vi "Example.vi"() -> ()   [LabVIEW 2017]
uses:
  Source/LAChatByText.vi
  Source/LAOnMessage.vi
  Source/LAOnChunk.vi
  Source/LAOnFunctionCall.vi
  Source/LAOnDone.vi
  Source/LAOnError.vi
  LiteAgentSDK.lvlib
panel:
  out "ToolReturn":cluster{"id":string, "result":variant}
  out "FunctionCall":T1
  out "AgentMessageChunkCompletions":T2
  out "AgentMessageChunkPart":T3
  out "AgentMessageChunkCommon":T4
  out "AgentMessageCompletions":T2
  out "AgentMessageContent":T5
  out "AgentMessageCommon":T4
  in  "Error In":errorcluster
  out "Error Output":errorcluster caption="Error Out"
  out "SessionId":string
  out "Version":string
  out "EventMessages":string
  out "Prompt":string
  out "AgentId":string
  out "ApiKey":string
  out "BaseUrl":string
  # "AgentMessage"
  # "AgentMessageChunk"
  # "FunctionCall & ToolReturn"
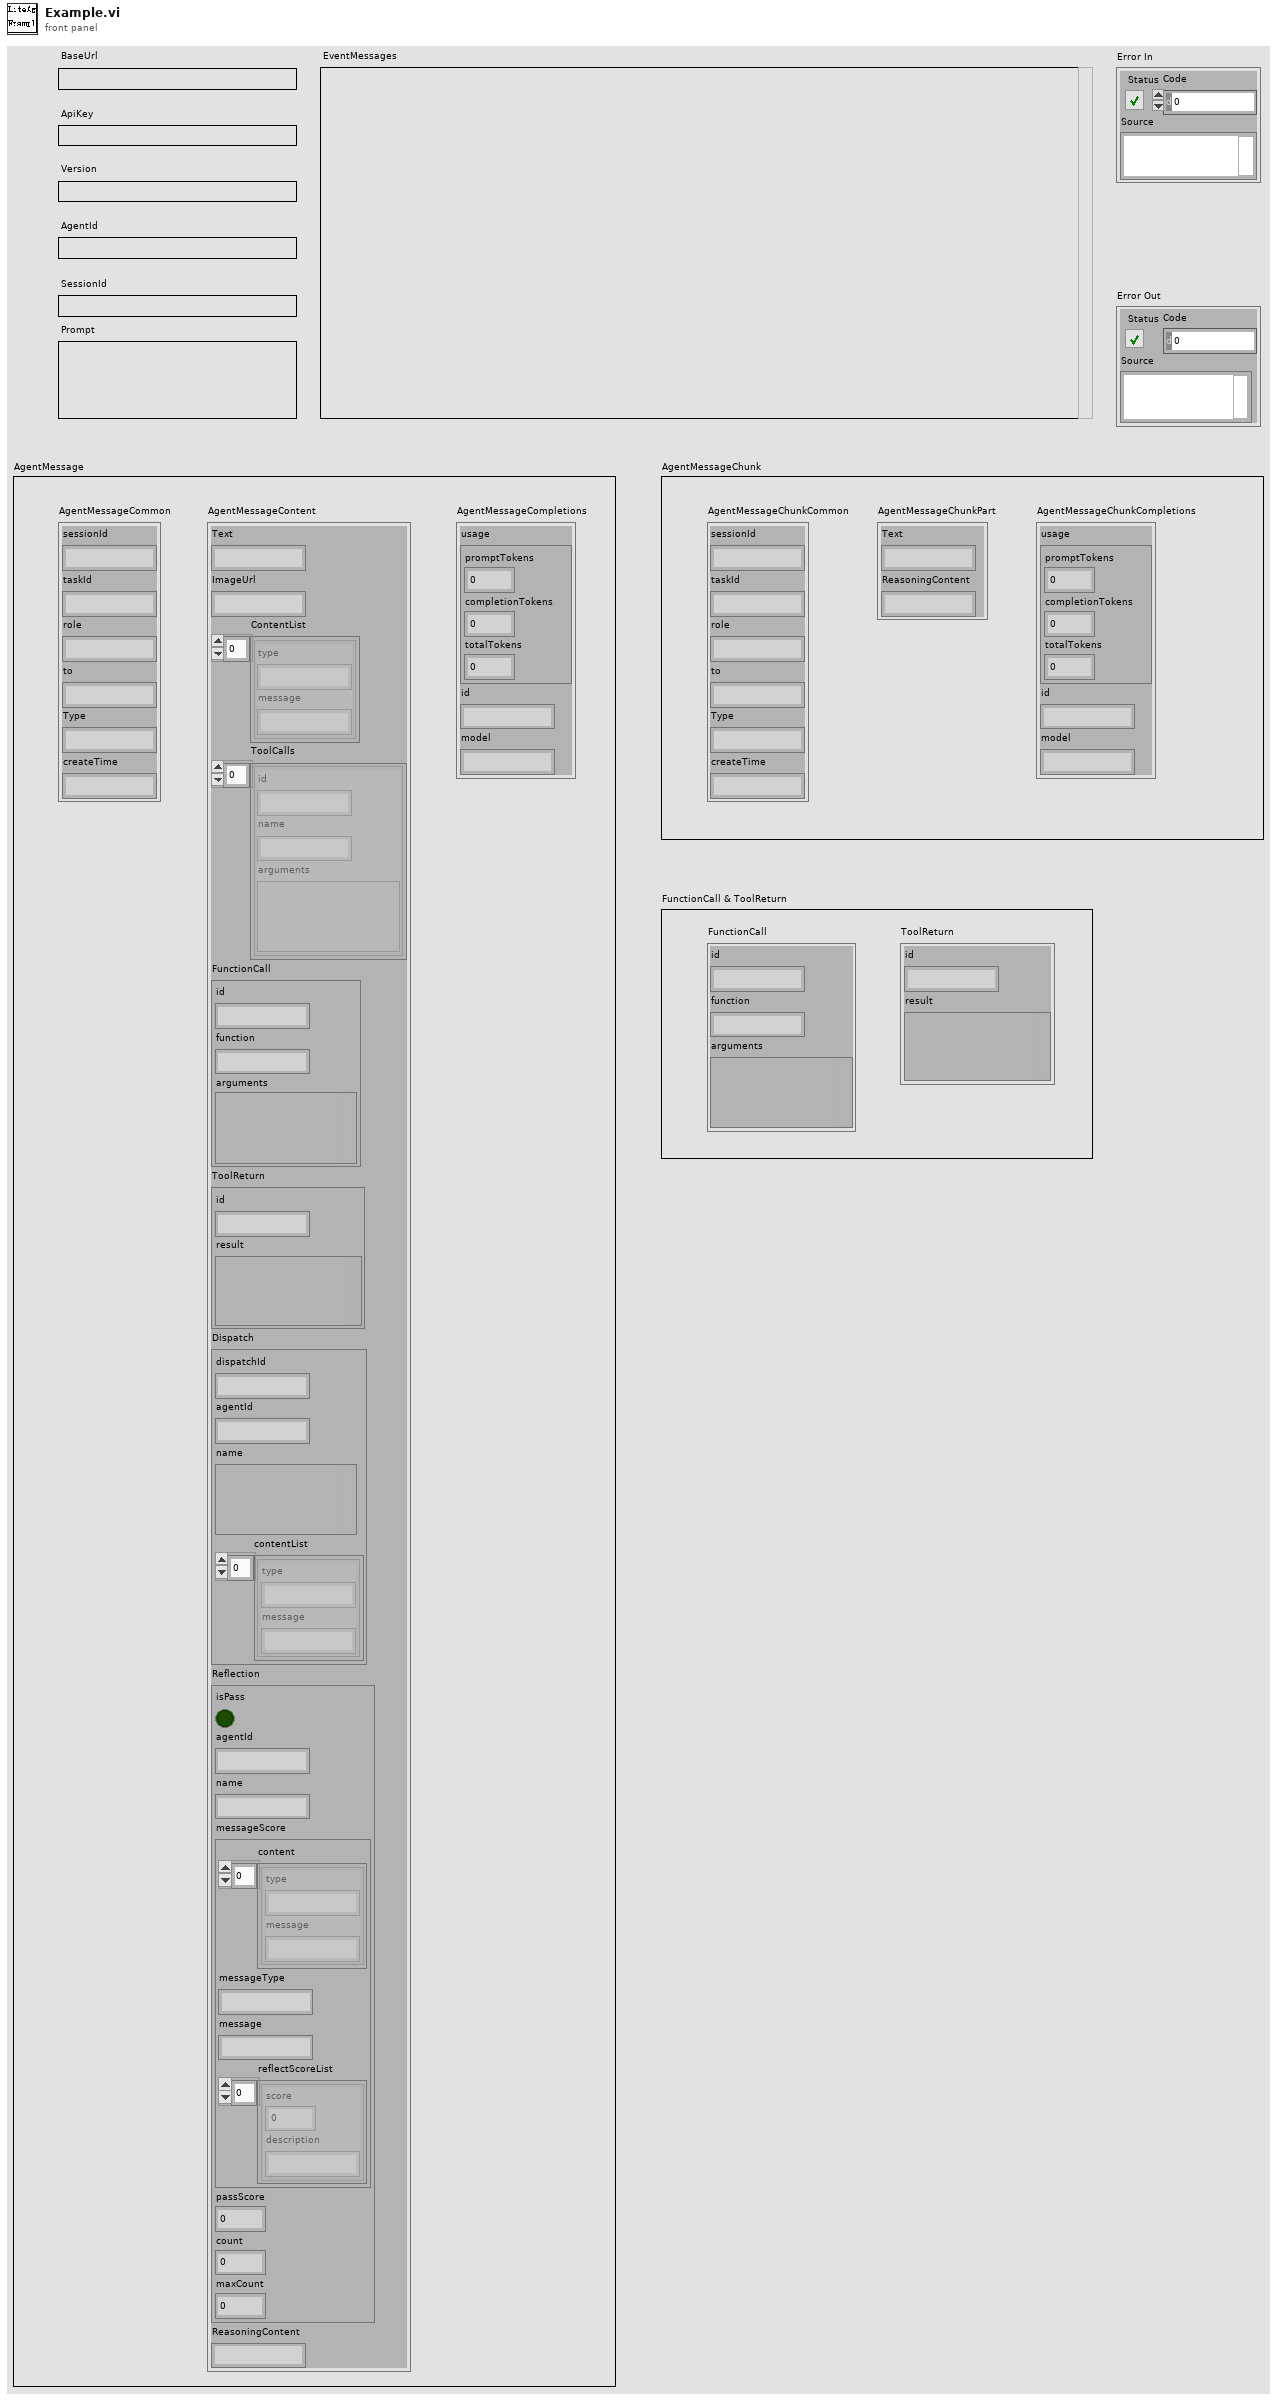
[diagram p1: front panel]
types:
  T1 = cluster{"id":string, "function":string, "arguments":variant}
  T2 = cluster{"usage":cluster{"promptTokens":i32, "completionTokens":i32, "totalTokens":i32}, "id":string, "model":string}
  T3 = cluster{"Text":string, "ReasoningContent":string}
  T4 = cluster{"sessionId":string, "taskId":string, "role":string, "to":string, "Type":string, "createTime":string}
  T5 = cluster{"Text":string, "ImageUrl":string, "ContentList":cluster{"type":string, "message":string}[], "ToolCalls":cluster{"id":string, "name":string, "arguments":variant}[], "FunctionCall":cluster{"id":string, "function":string, "arguments":variant}, "ToolReturn":cluster{"id":string, "result":variant}, "Dispatch":cluster{"dispatchId":string, "agentId":string, "name":variant, "contentList":cluster{"type":string, "message":string}[]}, "Reflection":cluster{"isPass":bool, "agentId":string, "name":string, "messageScore":cluster{"content":cluster{"type":string, "message":string}[], "messageType":string, "message":string, "reflectScoreList":cluster{"score":i32, "description":string}[]}, "passScore":i32, "count":i32, "maxCount":i32}, "ReasoningContent":string}
  T6 = cluster{"BaseUrl":string, "ApiKey":string, "LiteAgentSDK":refnum<k24>, "AgentId":string, "SessionId":string, "OnEventQueue":refnum<queue>, "CurrEventJson":variant}
  T7 = cluster{"sessionId":string, "taskId":string, "role":string, "to":string, "type":string, "content":variant, "completions":variant, "createTime":string}
  T8 = cluster{"sessionId":string, "taskId":string, "role":string, "to":string, "type":string, "part":variant, "completions":variant, "createTime":string}
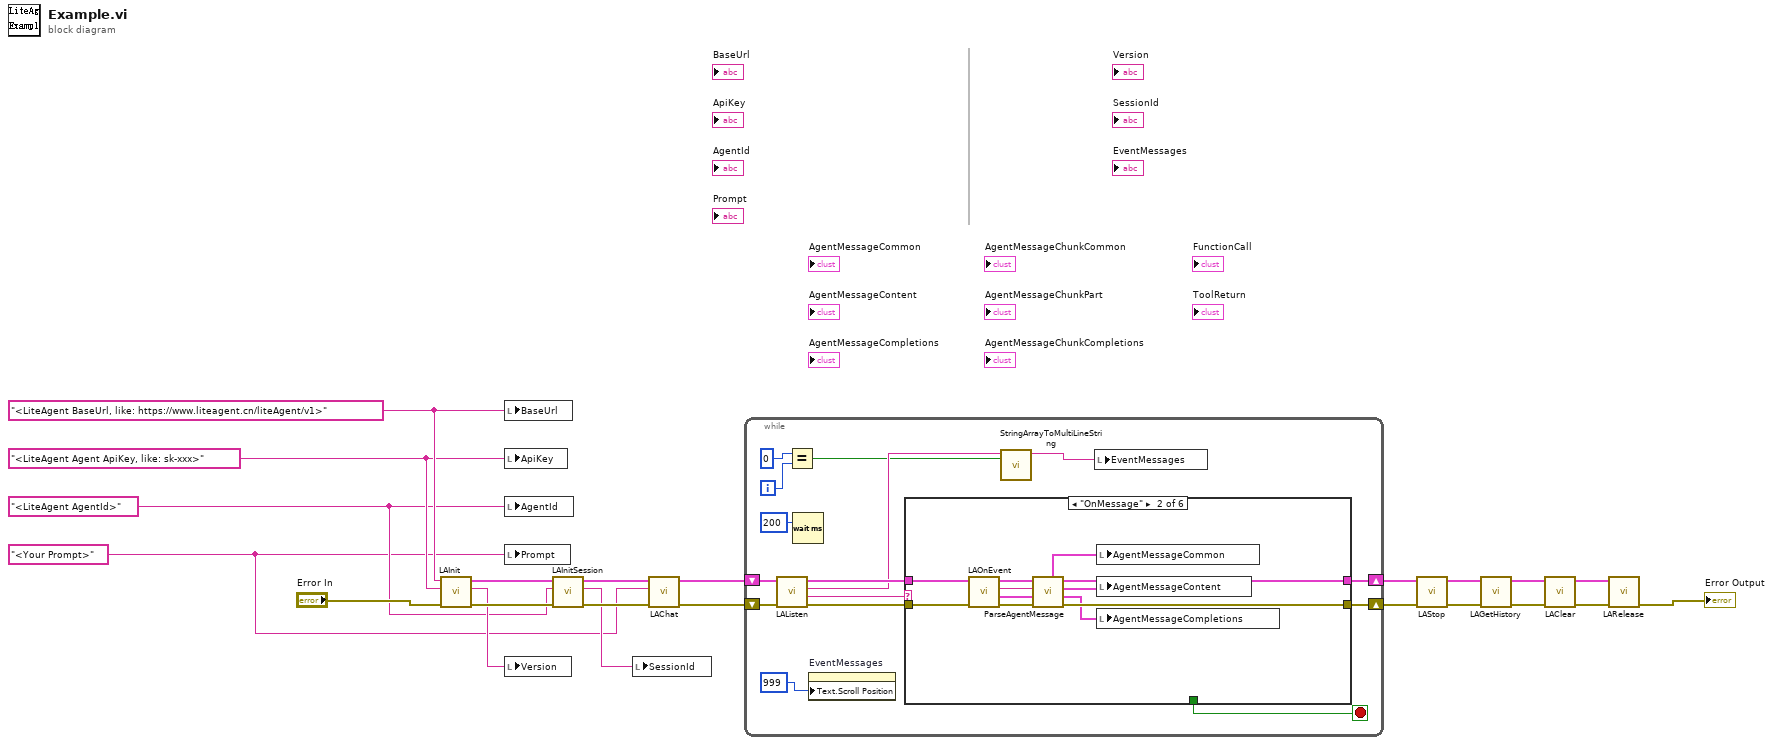
[diagram p0: block diagram]
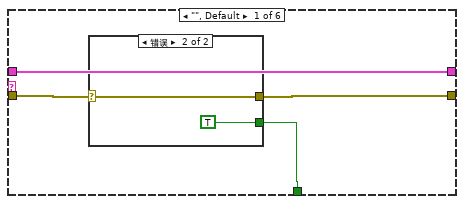
[diagram p2: hidden frame]
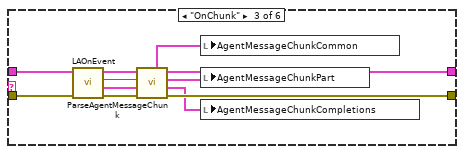
[diagram p4: hidden frame]
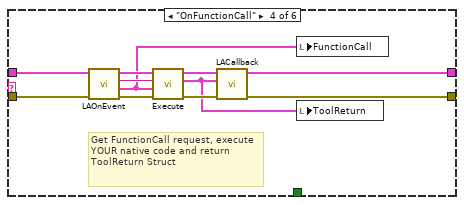
[diagram p5: hidden frame]
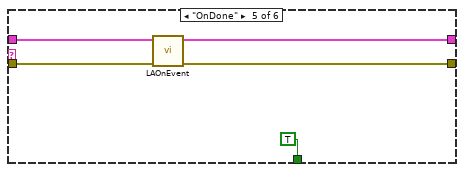
[diagram p6: hidden frame]
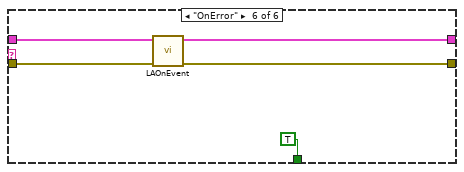
[diagram p7: hidden frame]
diagram:
  w1 = "<Your Prompt>"
  w2 = "<LiteAgent AgentId>"
  w3 = "<LiteAgent Agent ApiKey, like: sk-xxx>"
  w4 = "<LiteAgent BaseUrl, like: https://www.liteagent.cn/liteAgent/v1>"
  n1 = call "LAInit.vi"("Error Input"="Error In", "ApiKey"=w3, "BaseUrl"=w4) -> ("Error Output"=w10:errorcluster, "Version"=w7:string, "LiteAgent"=w9:T6)  [unwired: 6 in]
  n2 = local write "BaseUrl"(w4) -> ()
  n3 = local write "ApiKey"(w3) -> ()
  n4 = local write "AgentId"(w2) -> ()
  n5 = local write "Prompt"(w1) -> ()
  n6 = local write "Version"(w7) -> ()
  n7 = call "LAInitSession.vi"("Error In"=w10, "AgentId"=w2, "LiteAgent In"=w9) -> ("Error Out"=w12:errorcluster, "SessionId"=w8:string, "LiteAgent Out"=w11:T6)  [unwired: 6 in]
  n8 = local write "SessionId"(w8) -> ()
  n9 = call-poly "LAChat.vi"("Error In"=w12, "Message"=w1, "LiteAgent In"=w11) -> ("Error Out"=w14:errorcluster, "LiteAgent Out"=w13:T6)  [unwired: 7 in]
  n10 = while {
    shift-right: [w33] -> w15
    shift-left: w13 -> [w37]
    shift-right: [w32] -> w16
    shift-left: w14 -> [w36]
    i -> [w27]
    stop <- w28 stop-if-true
    n11 = call "LAListen.vi"("Error In"=w36, "LiteAgent In"=w37) -> ("Error Out"=w34:errorcluster, "Type"=w31:string, "EventJson"=w29:string, "LiteAgent Out"=w35:T6)  [unwired: 6 in]
    n12 = Equal?(x=0, y=w27) -> (x = y?=w26:bool)
    n13 = Wait (ms)(milliseconds to wait=u32 200 ("等待时间（毫秒）")) -> ()  [unwired: 1 out]
    n14 = property on="EventMessages" class="Str"("Text.Scroll Position"=u32 999 ("文本.滚动条位置")) -> ()  [unwired: 2 in, 2 out]
    n15 = case shown="\"OnMessage\"" w31 {
      tunnel: w35 -> [w41 w55 w66 w75 w81 w86]
      tunnel: w34 -> [w40 w54 w65 w74 w80 w85]
      tunnel: [w38 _ _ _ TRUE TRUE] -> w28
      tunnel: [w41 w48 w62 w76 w78 w84] -> w33
      tunnel: [w39 w52 w61 w77 w79 w83] -> w32
      frame "", Default {
        n16 = case shown="错误" w40 {
          selector: w40 -> [w42 w44]
          tunnel: [w42 w44] -> w39
          tunnel: [_ TRUE] -> w38
          frame No Error {
          }
          frame Error {
          }
        }
      }
      frame "OnMessage" {
        n17 = call-poly "LAOnEvent.vi"("Error In"=w54, "LiteAgent In"=w55) -> ("Error Out"=w53:errorcluster, "AgentMessage"=w49:T7, "SessionId"=w50:string, "LiteAgent Out"=w51:T6)  [unwired: 6 in]
        n18 = call "ParseAgentMessage.vi"("Error In"=w53, "AgentMessage"=w49, "SessionId"=w50, "LiteAgent In"=w51) -> ("Error Out"=w52:errorcluster, "Completions"=w45:T2, "Content"=w46:T5, "LiteAgent Out"=w48:T6, "Common"=w47:T4)  [unwired: 3 in]
        n19 = local write "AgentMessageCommon"(w47) -> ()
        n20 = local write "AgentMessageContent"(w46) -> ()
        n21 = local write "AgentMessageCompletions"(w45) -> ()
      }
      frame "OnChunk" {
        n22 = call-poly "LAOnEvent.vi"("Error In"=w65, "LiteAgent In"=w66) -> ("Error Out"=w60:errorcluster, "AgentMessageChunk"=w59:T8, "SessionId"=w64:string, "LiteAgent Out"=w63:T6)  [unwired: 6 in]
        n23 = call "ParseAgentMessageChunk.vi"("Error In"=w60, "AgentMessage"=w59, "SessionId"=w64, "LiteAgent In"=w63) -> ("Error Out"=w61:errorcluster, "Completions"=w56:T2, "Part"=w57:T3, "LiteAgent Out"=w62:T6, "Common"=w58:T4)  [unwired: 3 in]
        n24 = local write "AgentMessageChunkCommon"(w58) -> ()
        n25 = local write "AgentMessageChunkPart"(w57) -> ()
        n26 = local write "AgentMessageChunkCompletions"(w56) -> ()
      }
      frame "OnFunctionCall" {
        # "Get FunctionCall request, execute YOUR native code and return ToolReturn Struct"
        n27 = call-poly "LAOnEvent.vi"("Error In"=w74, "LiteAgent In"=w75) -> ("Error Out"=w73:errorcluster, "FunctionCall"=w67:T1, "SessionId"=w69:string, "LiteAgent Out"=w71:T6)  [unwired: 6 in]
        n28 = call "Execute.vi"("Error Input"=w73, "FunctionCall"=w67, "SessionId"=w69, "LiteAgent In"=w71) -> ("Error Output"=w72:errorcluster, "ToolReturn"=w68:cluster{"id":string, "result":variant}, "LiteAgent Out"=w70:T6)  [unwired: 5 in]
        n29 = call "LACallback.vi"("Error In"=w72, "ToolReturn"=w68, "LiteAgent In"=w70) -> ("Error Out"=w77:errorcluster, "LiteAgent Out"=w76:T6)  [unwired: 7 in]
        n30 = local write "FunctionCall"(w67) -> ()
        n31 = local write "ToolReturn"(w68) -> ()
      }
      frame "OnDone" {
        n32 = call-poly "LAOnEvent.vi"("Error In"=w80, "LiteAgent In"=w81) -> ("Error Out"=w79:errorcluster, "LiteAgent Out"=w78:T6)  [unwired: 8 in]
      }
      frame "OnError" {
        n33 = call-poly "LAOnEvent.vi"("Error In"=w85, "LiteAgent In"=w86) -> ("Error Out"=w83:errorcluster, "LiteAgent Out"=w84:T6)  [unwired: 7 in, 1 out]
      }
    }
    n34 = call "StringArrayToMultiLineString.vi"("Reset"=w26, "String"=w29) -> ("MultiLineString"=w30:string)  [unwired: 9 in]
    n35 = local write "EventMessages"(w30) -> ()
  }
  n36 = call "LAStop.vi"("Error In"=w16, "LiteAgent In"=w15) -> ("Error Out"=w18:errorcluster, "LiteAgent Out"=w17:T6)  [unwired: 8 in]
  n37 = call "LAGetHistory.vi"("Error Input"=w18, "LiteAgent In"=w17) -> ("Error Output"=w19:errorcluster, "LiteAgent Out"=w20:T6)  [unwired: 7 in, 1 out]
  n38 = call "LAClear.vi"("Error Input"=w19, "LiteAgent In"=w20) -> ("Error Output"=w21:errorcluster, "LiteAgent Out"=w22:T6)  [unwired: 8 in]
  n39 = call "LARelease.vi"("Error Input"=w21, "LiteAgent In"=w22) -> ("Error Output"=→"Error Output":errorcluster)  [unwired: 9 in]
